vi "Test Oxford ID and Read.vi"() -> ()   [LabVIEW 2016]
panel:
  out "read buffer":string
  in  "VISA resource name":refnum<visa-resource-name>="COM1"
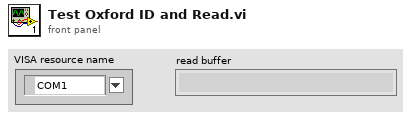
[diagram p1: front panel]
types:
  T1 = typedef "Device type.ctl" = enum16{"NONE", "Neocera 21", "LakeShore 335", "LakeShore 336", "LakeShore 340", "LkShr 340 chA&B", "LakeShore 370", "SRS 850", "SRS 830", "LR 700", "EG&G 5302", "EG&G 7260", "EG&G 7280", "AH 2500", "Keithley meter", "Keithley electrometer", "Keithley 182", "HP 5385", "HP 53181", "HP 53132", "ITC503", "IPS120", "Oxford Mercury IPS", "Oxford PS", "Test", "DC Facility Magnet", "Cryomagnetics PS", "Keithley 2400", "Keithley current source", "Cryo-Con 22C", "HP87NN", "HP4395A", "Agilent 34410A"}
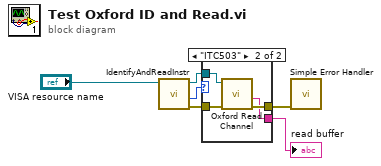
[diagram p0: block diagram]
diagram:
  n1 = call "IdentifyAndReadInstr.vi"("VISA Resource Name"="VISA resource name") -> ("error out"=w3:errorcluster, "Instrument"=w5:T1, "VISA Resource Name Out"=w4:refnum<visa-resource-name>)  [unwired: 7 in, 1 out]
  n2 = case shown="\"ITC503\"" w5 {
    tunnel: w4 -> [_ w11]
    tunnel: w3 -> [w7 w10]
    tunnel: [w7 w9] -> w2
    tunnel: [_ w8] -> w1
    frame "NONE", Default {
    }
    frame "ITC503" {
      n3 = call "Oxford Read Channel.vi"("error in (no error)"=w10, "VISA resource name"=w11) -> ("error out"=w9:errorcluster, "read buffer"=w8:string)  [unwired: 6 in, 2 out]
    }
  }
  "read buffer" <- w1
  n4 = call <vilib>:"Simple Error Handler.vi"("error in (no error)"=w2) -> ()  [unwired: 4 in, 5 out]
